vi "stealBallSkill.vi"(6 "Field":refnum<class "Field.lvclass">, 8 "error in (no error)":errorcluster, 9 "Ball":refnum<class "Ball.lvclass">, 10 "Robot":refnum<class "Robot.lvclass">, 11 "StealBallSkill in":refnum<class "StealBallSkill.lvclass">) -> (0 "error out":errorcluster, 2 "Robot out":refnum<class "Robot.lvclass">, 3 "StealBallSkill out":refnum<class "StealBallSkill.lvclass">)   [LabVIEW 2023, in "StealBallSkill.lvclass"]
uses:
  StealBallSkill.lvclass
  Ball_class/Ball.lvclass
  Field_class/Field.lvclass
  Robot_class/Robot.lvclass
  Robot_class/Robot.lvclass/Robot.ctl
  Robot_class/Write dest_x.vi
  Robot_class/Write dest_y.vi
  Robot_class/Write dest_orientation.vi
  Utilities_class/Utilities.lvclass
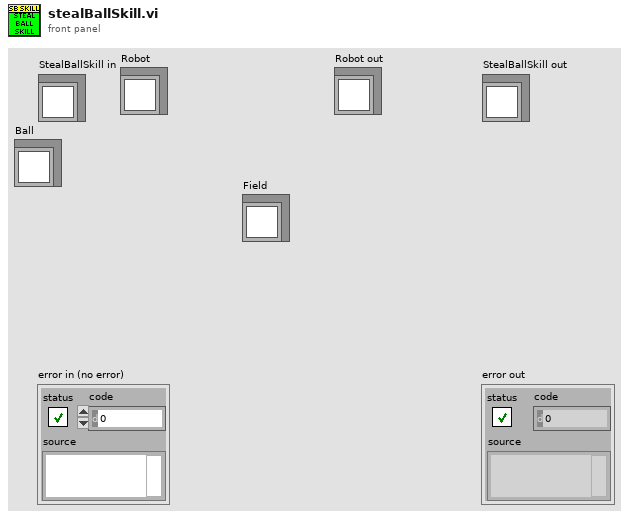
[diagram p1: front panel]
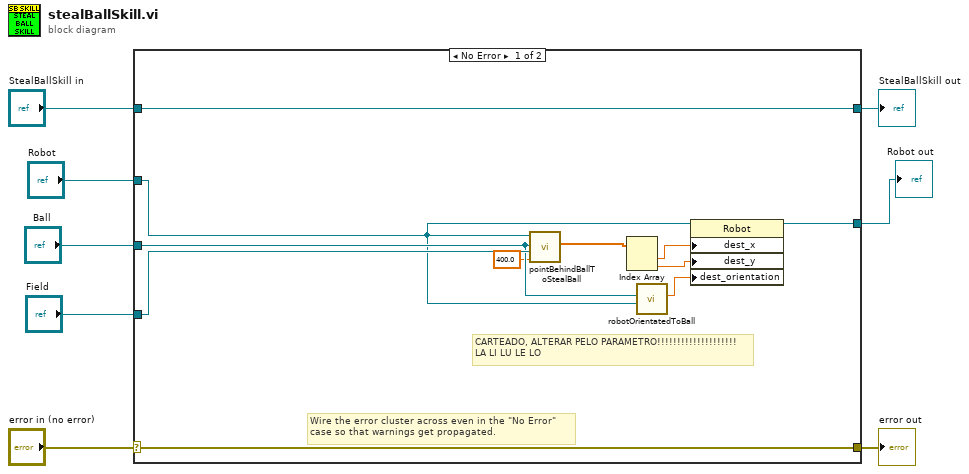
[diagram p0: block diagram]
diagram:
  n1 = case shown="No Error" "error in (no error)" {
    selector: "error in (no error)" -> [w18 w21]
    tunnel: [w18 w21] -> w7
    tunnel: [w19 w20] -> w5
    tunnel: "StealBallSkill in" -> [w19 w20]
    tunnel: "Ball" -> [w12 _]
    tunnel: "Field" -> [w17 _]
    tunnel: "Robot" -> [w11 _]
    tunnel: [w10 _] -> w1
    frame No Error {
      # "CARTEADO, ALTERAR PELO PARAMETRO!!!!!!!!!!!!!!!!!!!!\nLA LI LU LE LO"
      # "Wire the error cluster across even in the \"No Error\"\ncase so that warnings get propagated."
      n2 = call "pointBehindBallToStealBall.vi"("distanceBehindBallToStealBall"=400.0, "Field"=w17, "Ball"=w12, "Robot in"=w11) -> ("pointBehindBall"=w13:dbl[])  [unwired: 7 in]
      n3 = Index Array(array=w13) -> (element #1=w16:dbl, element #2=w15:dbl)  [unwired: 2 in]
      n4 = call "robotOrientatedToBall.vi"("Robot"=w11, "BallRef"=w12) -> ("Orientation"=w14:dbl)  [unwired: 7 in, 2 out]
      n5 = property class="Robot"(reference=w11, "dest_x"=w16, "dest_y"=w15, "dest_orientation"=w14) -> (reference out=w10:refnum<class "Robot.lvclass">)  [unwired: 1 in, 1 out]
    }
    frame Error {
    }
  }
  "error out" <- w7
  "StealBallSkill out" <- w5
  "Robot out" <- w1
